vi "File Writing Example.vi"() -> ()   [LabVIEW 2014]
panel:
  in  "File Format":enum16{"CSV", "Binary", "HDF5", "TDMS"}(ring)
  out "Time Stamp":timestamp
  in  "Dataset (HDF5) or Group (TDMS)":string="MyData"
  in  "File Path":path
  in  "Comment":string="Testing file writing"
  in  "tf (s)":dbl=3600.0
  out "XY Graph":cluster{dbl[], dbl[]}[](graph)
  in  "Tf":dbl=5.0
  in  "T0":dbl=95.0
  in  "dt":dbl=0.1
  in  "k":dbl=0.0009
  # "Cooling Params"
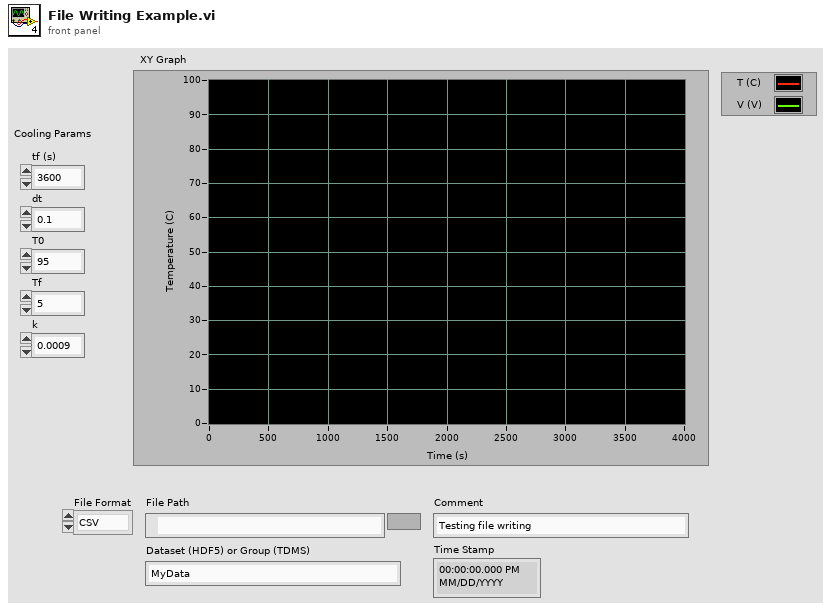
[diagram p1: front panel]
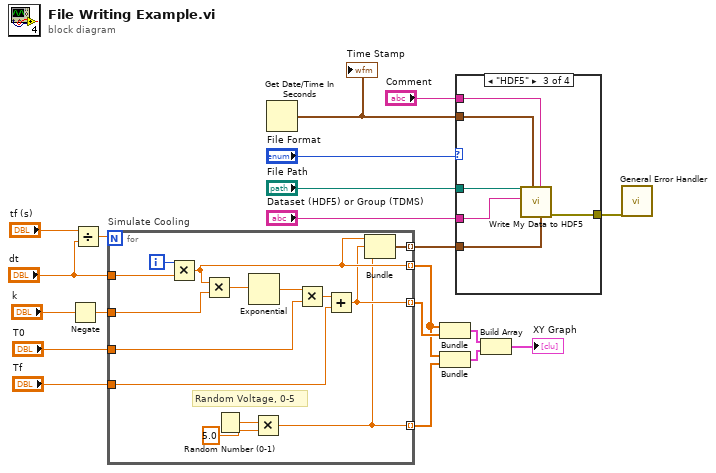
[diagram p0: block diagram]
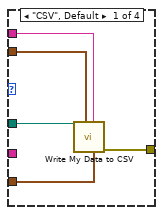
[diagram p2: hidden frame]
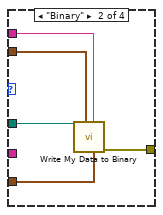
[diagram p3: hidden frame]
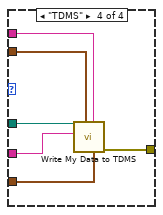
[diagram p4: hidden frame]
diagram:
  n1 = Negate(x="k") -> (-x=w12:dbl)
  n2 = Divide(x="tf (s)", y="dt") -> (x/y=w13:dbl)
  n3 = for "Simulate Cooling" {
    N: w13 -> [_]
    tunnel: "dt" -> [w30]
    tunnel: w12 -> [w29]
    tunnel: "T0" -> [w28]
    tunnel: "Tf" -> [w27]
    tunnel: [w24] -> w11 mode=indexing
    tunnel: [w23] -> w14 mode=indexing
    tunnel: [w22] -> w10 mode=indexing
    tunnel: [w21] -> w3 mode=indexing
    i -> [w34]
    # "Random Voltage, 0-5"
    n4 = Multiply(x=w34, y=w30) -> (x*y=w24:dbl)
    n5 = Multiply(x=w24, y=w29) -> (x*y=w33:dbl)
    n6 = Random Number (0-1)() -> (number: 0 to 1=w26:dbl)
    n7 = Exponential(1:w33) -> (0:w32:dbl)
    n8 = Multiply(x=w26, y=5.0) -> (x*y=w22:dbl)
    n9 = Multiply(x=w32, y=w28) -> (x*y=w31:dbl)
    n10 = Add(x=w31, y=w27) -> (x+y=w23:dbl)
    n11 = Bundle(w24, w23, w22) -> (w21:cluster{dbl, dbl, dbl})  [unwired: 1 in]
  }
  n12 = Get Date/Time In Seconds() -> (seconds since 1Jan1904=w5:timestamp)
  "Time Stamp" <- w5
  n13 = Bundle(w11, w14) -> (w9:cluster{dbl[], dbl[]})  [unwired: 1 in]
  n14 = Bundle(w11, w10) -> (w8:cluster{dbl[], dbl[]})  [unwired: 1 in]
  n15 = case shown="\"HDF5\"" "File Format" {
    tunnel: "File Path" -> [w39 w44 w50 w56]
    tunnel: w5 -> [w38 w43 w49 w55]
    tunnel: "Comment" -> [w37 w42 w48 w54]
    tunnel: w3 -> [w36 w41 w45 w53]
    tunnel: [w35 w40 w47 w52] -> w2
    tunnel: "Dataset (HDF5) or Group (TDMS)" -> [_ _ w46 w51]
    frame "CSV", Default {
      n16 = call "Write My Data to CSV.vi"("Data"=w36, "Comment"=w37, "Time Stamp"=w38, "file path"=w39) -> ("error out"=w35:errorcluster)  [unwired: 7 in]
    }
    frame "Binary" {
      n17 = call "Write My Data to Binary.vi"("Data"=w41, "Comment"=w42, "Time Stamp"=w43, "file path"=w44) -> ("error out"=w40:errorcluster)  [unwired: 7 in]
    }
    frame "HDF5" {
      n18 = call "Write My Data to HDF5.vi"("Data"=w45, "Comment"=w48, "Time Stamp"=w49, "Dataset Path"=w46, "file path"=w50) -> ("error out"=w47:errorcluster)  [unwired: 6 in]
    }
    frame "TDMS" {
      n19 = call "Write My Data to TDMS.vi"("Data"=w53, "Comment"=w54, "Time Stamp"=w55, "Dataset Path"=w51, "file path"=w56) -> ("error out"=w52:errorcluster)  [unwired: 6 in]
    }
  }
  n20 = Build Array(w9, w8) -> (→"XY Graph":cluster{dbl[], dbl[]}[])
  n21 = call <vilib>:"General Error Handler.vi"("error in (no error)"=w2) -> ()  [unwired: 10 in, 5 out]
